vi "Load Sequence.vi"(8 "error in (no error)":errorcluster, 9 "Skip File Dialog?(F)":bool, 10 "Browse path":path, 11 "Message List Elements":T1[](array[typedef])) -> (0 "error out":errorcluster, 3 "Uncompiled Sequence out":T2[](array[typedef]))   [LabVIEW 2020, in "Sequencer.lvlib"]
doc: "Load uncompiled sequence from a sequence file."
uses:
  Sequencer.lvlib
  Controls/Ctl_SequenceElement.ctl
  Controls/Ctl_SequenceControlElement.ctl
  PPL/HDH.Actor Framework.Core.Msg.lvlibp/Flex Msg/Controls/Ctl_Control Element.ctl
  Controls/Ctl_MessageListElement.ctl
  Sequencer Messages/Load Failure Msg/Load Failure Msg.lvclass
  PPL/HDH.Actor Framework.Core.Msg.lvlibp
  PPL/HDH.Data.Generic.lvlibp
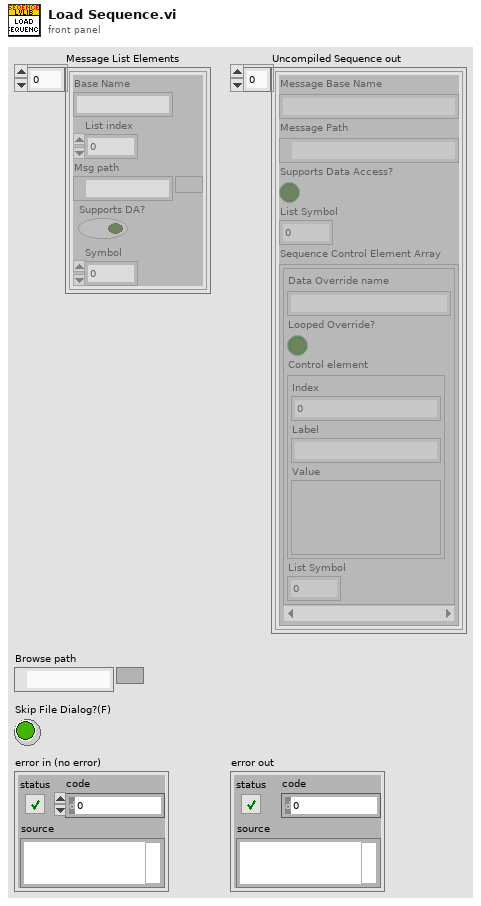
[diagram p1: front panel]
types:
  T1 = typedef "Sequencer.lvlib/Ctl_MessageListElement.ctl" = cluster{"Base Name":string, "List index":i32, "Msg path":path, "Supports DA?":bool, "Symbol":i32}
  T2 = typedef "Sequencer.lvlib/Ctl_SequenceElement.ctl" = cluster{"Message Base Name":string, "Message Path":path, "Supports Data Access?":bool, "List Symbol":i32, "Sequence Control Element Array":T3[]}
  T3 = typedef "Sequencer.lvlib/Ctl_SequenceControlElement.ctl" = cluster{"Data Override name":string, "Looped Override?":bool, "Control element":T4, "List Symbol":i32}
  T4 = typedef "HDH.Actor Framework.Core.Msg.lvlibp/Ctl_Control Element.ctl" = cluster{"Index":i32, "Label":string, "Value":variant}
  T5 = enum16{"open", "replace", "create", "open or create", "replace or create", "replace or create with confirmation"}
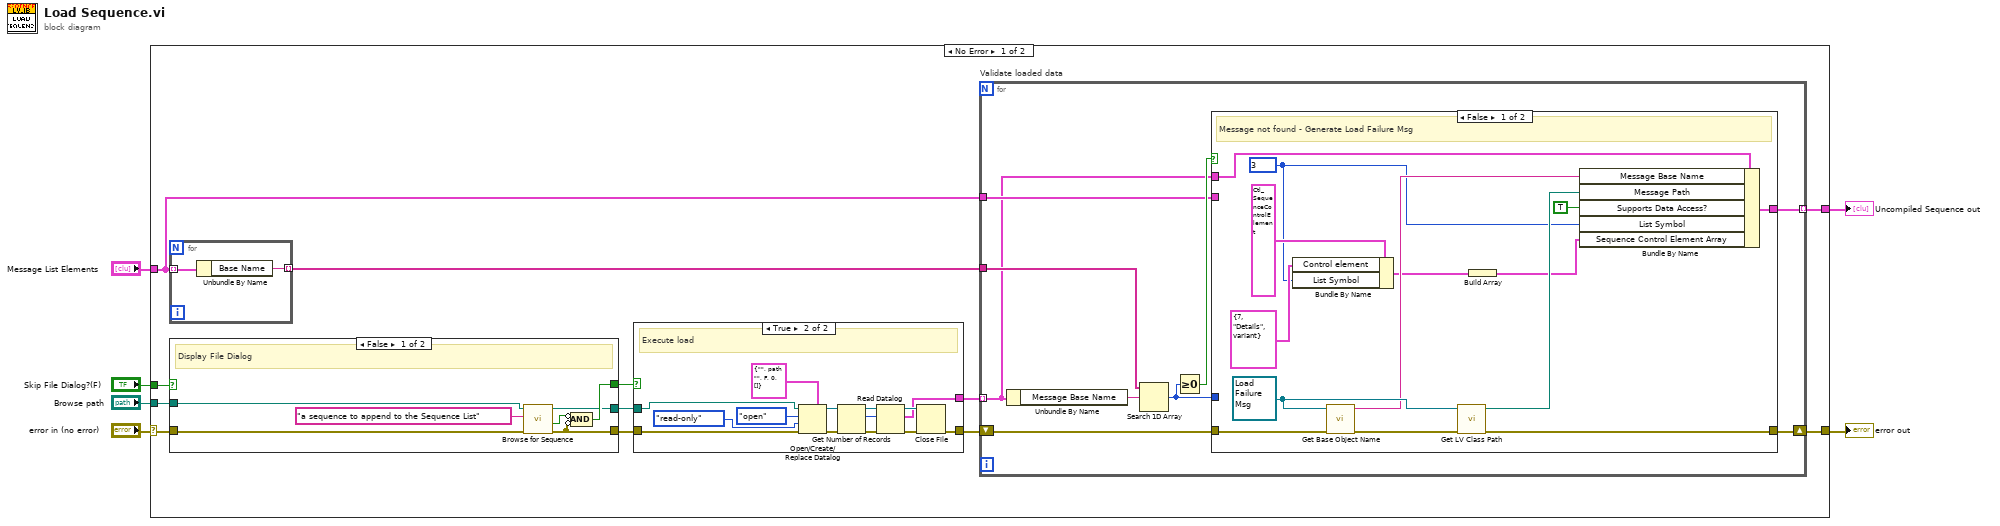
[diagram p0: block diagram]
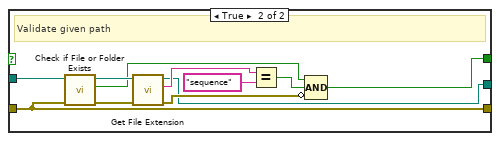
[diagram p2: hidden frame]
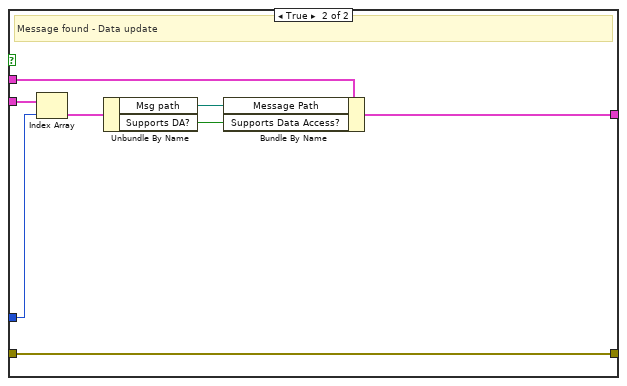
[diagram p3: hidden frame]
diagram:
  n1 = case shown="No Error" "error in (no error)" {
    selector: "error in (no error)" -> [w18 w85]
    tunnel: [w8 w85] -> w6
    tunnel: "Browse path" -> [w14 _]
    tunnel: [w10 _] -> w3
    tunnel: "Message List Elements" -> [w12 _]
    tunnel: "Skip File Dialog?(F)" -> [w7 _]
    frame No Error {
      n2 = for {
        tunnel: w12 -> [w69] mode=indexing
        tunnel: [w68] -> w13 mode=indexing
        n3 = Unbundle By Name(w69) -> ("Base Name"=w68:string)
      }
      n4 = case shown="False" w7 {
        tunnel: w18 -> [w23 w28]
        tunnel: [w21 w26] -> w17
        tunnel: [w19 w28] -> w16
        tunnel: [w25 w27] -> w15
        tunnel: w14 -> [w24 w36]
        frame False {
          # "Display File Dialog"
          n5 = call "Browse for Sequence.vi"("error in (no error)"=w23, "Caption (Browse for/Select concatenated)"="a sequence to append to the Sequence List" ("prompt"), "Browse start path"=w24) -> ("error out"=w19:errorcluster, "Cancelled?"=w20:bool, "File Path out"=w21:path)  [unwired: 6 in]
          n6 = Compound Arithmetic op=AND(invert w20, invert w19) -> (w25:bool)
        }
        frame True {
          # "Validate given path"
          n7 = call <vilib>:"Check if File or Folder Exists.vi"("error in (no error)"=w28, "path"=w36) -> ("error out"=w34:errorcluster, "file or folder exists?"=w31:bool, "dup path"=w35:path)  [unwired: 7 in]
          n8 = call <vilib>:"Get File Extension.vi"("error in (no error)"=w34, "file"=w35) -> ("error out"=w29:errorcluster, "lowercase file extension"=w33:string, "dup file"=w26:path)  [unwired: 5 in, 2 out]
          n9 = Equal?(x=w33, y="sequence" ("lowercase file extension")) -> (x = y?=w30:bool)
          n10 = Compound Arithmetic op=AND(w31, w30, invert w29) -> (w27:bool)
        }
      }
      n11 = case shown="True" w15 {
        tunnel: [w70 w81] -> w9
        tunnel: w16 -> [w70 w82]
        tunnel: w17 -> [_ w84]
        tunnel: [_ w73] -> w11
        frame False {
          # "Cancelled or error"
        }
        frame True {
          # "Execute load"
          n12 = Open/Create/Replace Datalog(5:T2 {"Message Base Name"="", "Message Path"=path "", "Supports Data Access?"=FALSE, "List Symbol"=0, "Sequence Control Element Array"=[]} ("element"), 8:w82, 9:enum16{"read/write", "read-only", "write-only"}."read-only" ("access (0:read/write)"), 10:T5."open" ("operation (0:open)"), 11:w84) -> (0:w78:errorcluster, 3:w79:refnum<k1>)  [unwired: 1 in, 1 out]
          n13 = Get Number of Records(4:w78, 7:w79) -> (0:w75:errorcluster, 2:w71:i64, 3:w77:refnum<k1>)
          n14 = Read Datalog(4:w75, 6:w71, 7:w77) -> (0:w74:errorcluster, 2:w73:T2[], 3:w76:refnum<k1>)
          n15 = Close File(refnum=w76, error in=w74) -> (error out=w81:errorcluster)  [unwired: 1 out]
        }
      }
      n16 = for "Validate loaded data" {
        tunnel: w11 -> [w40] mode=indexing
        tunnel: w13 -> [w45]
        tunnel: w12 -> [w42]
        tunnel: [w39] -> w10 mode=indexing
        shift-right: [w37] -> w8
        shift-left: w9 -> [w38]
        n17 = Unbundle By Name(w40) -> ("Message Base Name"=w44:string)
        n18 = Search 1D Array(1D array=w45, element=w44) -> (index of element=w41:i32)  [unwired: 1 in]
        n19 = Greater Or Equal To 0?(x=w41) -> (x >= 0?=w43:bool)
        n20 = case shown="False" w43 {
          tunnel: w42 -> [_ w67]
          tunnel: w41 -> [_ w66]
          tunnel: w40 -> [w53 w64]
          tunnel: [w47 w61] -> w39
          tunnel: w38 -> [w59 w60]
          tunnel: [w46 w60] -> w37
          frame False {
            w50 = 3
            w58 = refnum<class "Load Failure Msg.lvclass"> refnum ("Sequencer.lvlib:Load Failure Msg.lvclass")
            # "Message not found - Generate Load Failure Msg"
            n21 = Bundle By Name(cluster=T3 {"Data Override name"="", "Looped Override?"=FALSE, "Control element"={"Index"=0, "Label"="", "Value"=variant}, "List Symbol"=0} ("Sequence Control Element"), "Control element"=T4 {"Index"=7, "Label"="Details", "Value"=variant}, "List Symbol"=w50) -> (w49:T3)
            n22 = call "Get Base Object Name.vi"("error in (no error)"=w59, "Object in"=w58) -> ("error out"=w55:errorcluster, "Base class name"=w57:string)  [unwired: 8 in]
            n23 = call <vilib>:"Get LV Class Path.vi"("error in (no error)"=w55, "object"=w58) -> ("error out"=w46:errorcluster, "class path"=w56:path)  [unwired: 8 in]
            n24 = Build Array(w49) -> (w48:T3[])
            n25 = Bundle By Name(cluster=w53, "Message Base Name"=w57, "Message Path"=w56, "Supports Data Access?"=TRUE, "List Symbol"=w50, "Sequence Control Element Array"=w48) -> (w47:T2)
          }
          frame True {
            # "Message found - Data update"
            n26 = Index Array(array=w67, index=w66) -> (element=w65:T1)
            n27 = Unbundle By Name(w65) -> ("Msg path"=w63:path, "Supports DA?"=w62:bool)
            n28 = Bundle By Name(cluster=w64, "Message Path"=w63, "Supports Data Access?"=w62) -> (w61:T2)
          }
        }
      }
    }
    frame Error {
    }
  }
  "error out" <- w6
  "Uncompiled Sequence out" <- w3
